vi "多参校准读取.vi"(8 "Error in":errorcluster caption="Error in (no error)", 11 "站号":u16(ring)=10 items=["氨氮"=3, "水温"=9, "pH值"=10, "溶解氧"=11, "电导率"=12, "浊度"=13, "叶绿素a"=14, "藻密度"=15, "蓝绿藻"=16, "氧化还原电位"=17, "溶解氧%"=18, "盐度"=19]) -> (0 "error out":errorcluster, 2 "B":dbl caption="校准值B:", 3 "K":dbl caption="校准值K:")   [LabVIEW 2016, in "斯坦道多参数.lvlib"]
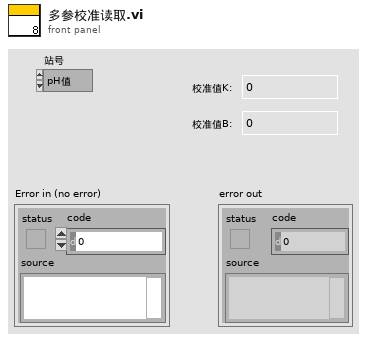
[diagram p1: front panel]
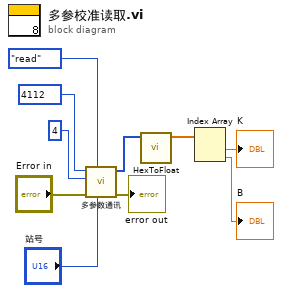
[diagram p0: block diagram]
diagram:
  n1 = call "多参数通讯.vi"("Slave ID"="站号", "STEP"=enum16{"open", "read", "write", "close"}."read", "Error in"="Error in", "quantity"=u16 4, "starting address"=u16 4112) -> ("error out"=→"error out":errorcluster, "Registers"=w8:u16[])  [unwired: 4 in, 1 out]
  n2 = call "HexToFloat.vi"("数组"=w8) -> ("FLOAT"=w7:sgl[])  [unwired: 10 in]
  n3 = Index Array(array=w7) -> (element #1=→"K":sgl, element #2=→"B":sgl)  [unwired: 2 in]
